vi "createCheese.vi"(8 "error in (no error)":errorcluster, 11 "ChicagoPizzaIngredientFactory in":refnum<class "ChicagoPizzaIngredientFactory.lvclass">) -> (0 "error out":errorcluster, 2 "Ingredients":string, 3 "ChicagoPizzaIngredientFactory out":refnum<class "ChicagoPizzaIngredientFactory.lvclass">)   [LabVIEW 2013, in "ChicagoPizzaIngredientFactory.lvclass"]
uses:
  ChicagoPizzaIngredientFactory.lvclass
  ChicagoPizzaIngredientFactory.lvclass/ChicagoPizzaIngredientFactory.ctl
  Cheese.lvclass/Cheese.lvclass
panel:
  # "產出起司"
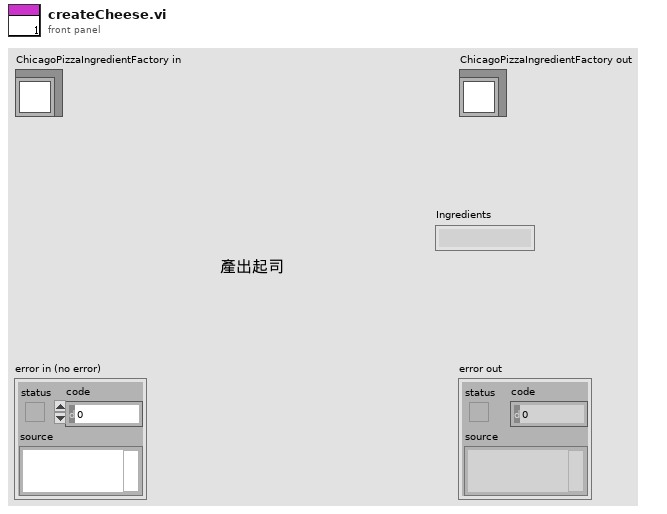
[diagram p1: front panel]
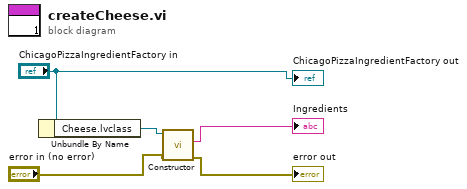
[diagram p0: block diagram]
diagram:
  n1 = Unbundle By Name("ChicagoPizzaIngredientFactory in") -> ("Cheese.lvclass"=w4:refnum<class "Cheese.lvclass">)
  n2 = call-dynamic "Constructor.vi"("error in (no error)"="error in (no error)", "Cheese in"=w4) -> ("error out"=→"error out":errorcluster, "Ingredients"=→"Ingredients":string)  [unwired: 7 in, 1 out]
  "ChicagoPizzaIngredientFactory out" <- "ChicagoPizzaIngredientFactory in"
